vi "PlotSubArray.vi"(8 "Time Step (s)":dbl, 9 "Plot Last x Seconds":dbl, 10 "Iteration":i32, 11 "Array":dbl[](array[numeric])) -> (0 "Sub Array":dbl[](array[numeric]), 3 "Time Offset":dbl)   [LabVIEW 2017]
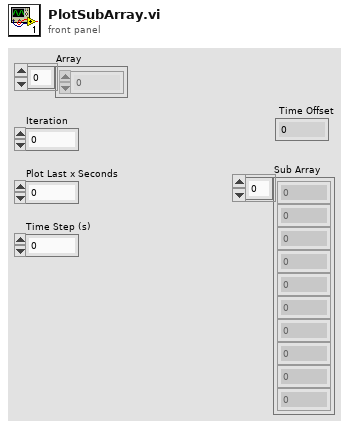
[diagram p1: front panel]
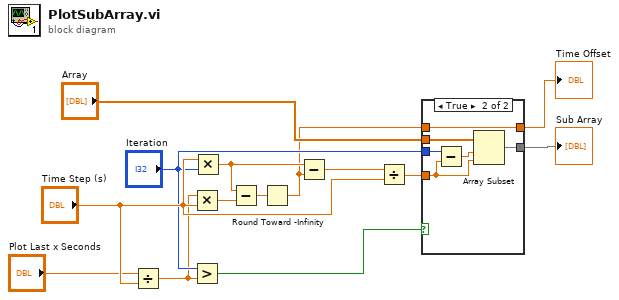
[diagram p0: block diagram]
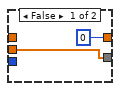
[diagram p2: hidden frame]
diagram:
  n1 = Divide(x="Plot Last x Seconds", y="Time Step (s)") -> (x/y=w6:dbl)
  n2 = Multiply(x=w6, y="Time Step (s)") -> (x*y=w10:dbl)
  n3 = Greater?(x="Iteration", y=w6) -> (0:w7:bool)
  n4 = Multiply(x="Time Step (s)", y="Iteration") -> (x*y=w12:dbl)
  n5 = Subtract(x=w12, y=w10) -> (x-y=w2:dbl)
  n6 = Round Toward -Infinity(1:w2) -> (0:w1:dbl)
  n7 = Subtract(x=w12, y=w1) -> (x-y=w3:dbl)
  n8 = Divide(x=w3, y="Time Step (s)") -> (x/y=w14:dbl)
  n9 = case shown="True" w7 {
    tunnel: "Array" -> [w16 w22]
    tunnel: [w16 w21] -> w4
    tunnel: "Iteration" -> [_ w19]
    tunnel: [0 w17] -> w11
    tunnel: w14 -> [_ w18]
    tunnel: w1 -> [_ w17]
    frame False {
    }
    frame True {
      n10 = Subtract(x=w19, y=w18) -> (x-y=w20:dbl)
      n11 = Array Subset(array=w22, index=w20, length=w18) -> (w21:dbl[])
    }
  }
  "Sub Array" <- w4
  "Time Offset" <- w11
